vi "Apply Config.vi"(8 "error in (no error)":errorcluster, 11 "GaugeIndicator in":refnum<class "GaugeIndicator.lvclass">) -> (0 "error out":errorcluster, 3 "GaugeIndicator out":refnum<class "GaugeIndicator.lvclass">)   [LabVIEW 2020, in "VolatusGUIElements.lvlib" / "GaugeIndicator.lvclass"]
uses:
  GaugeIndicator.lvclass
  GaugeIndicator.lvclass/GaugeIndicator.ctl
  Value Source.ctl
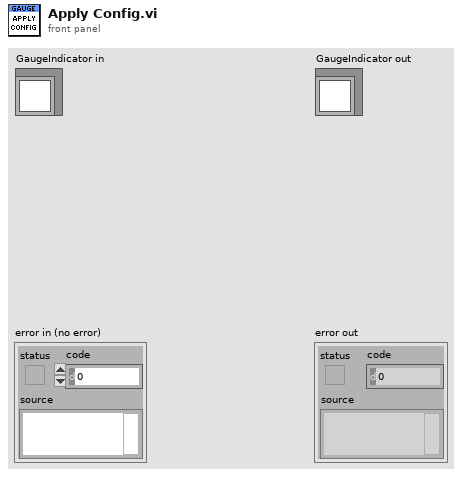
[diagram p1: front panel]
types:
  T1 = typedef "VolatusGUIElements.lvlib/GaugeIndicator.lvclass/Value Source.ctl" = enum16{"Constant", "Channel"}
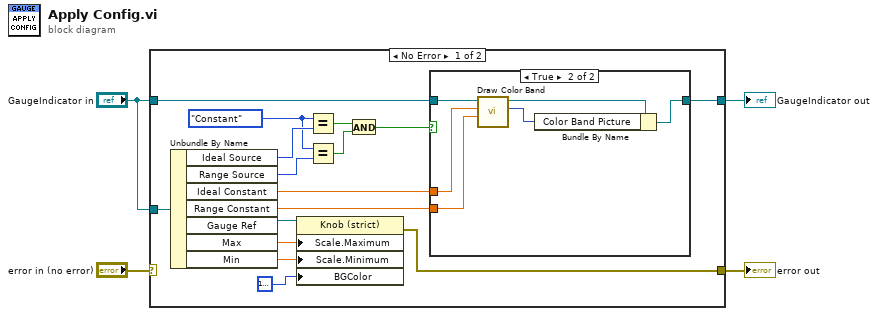
[diagram p0: block diagram]
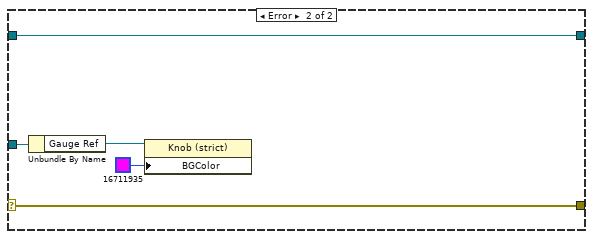
[diagram p3: hidden frame]
diagram:
  n1 = case shown="No Error" "error in (no error)" {
    selector: "error in (no error)" -> [_ w30]
    tunnel: "GaugeIndicator in" -> [w20 w32]
    tunnel: [w15 w30] -> w3
    tunnel: "GaugeIndicator in" -> [w9 w28]
    tunnel: [w5 w28] -> w1
    frame No Error {
      w12 = Value_Source."Constant" ("x")
      n2 = Unbundle By Name(w20) -> ("Ideal Source"=w14:T1, "Range Source"=w13:T1, "Ideal Constant"=w6:dbl, "Range Constant"=w7:dbl, "Gauge Ref"=w19:refnum<vi>, "Max"=w18:dbl, "Min"=w17:dbl)
      n3 = property class="Knob (strict)"(reference=w19, "Scale.Maximum"=w18, "Scale.Minimum"=w17, "BGColor"=u32 16777216 ("Housing Colors:BG Color")) -> (error out=w15:errorcluster)  [unwired: 1 in, 1 out]
      n4 = Equal?(x=w12, y=w14) -> (x = y?=w11:bool)
      n5 = Equal?(x=w12, y=w13) -> (x = y?=w10:bool)
      n6 = And(x=w11, y=w10) -> (x .and. y?=w8:bool)
      n7 = case shown="True" w8 {
        tunnel: w9 -> [w21 w27]
        tunnel: w7 -> [_ w25]
        tunnel: w6 -> [_ w26]
        tunnel: [w21 w22] -> w5
        frame False {
        }
        frame True {
          n8 = call "Draw Color Band.vi"("Range"=w25, "Ideal"=w26, "GaugeIndicator in"=w27) -> ("Color Band"=w23:picture, "GaugeIndicator out"=w24:refnum<class "GaugeIndicator.lvclass">)  [unwired: 6 in, 1 out]
          n9 = Bundle By Name(cluster=w24, "Color Band Picture"=w23) -> (w22:refnum<class "GaugeIndicator.lvclass">)
        }
      }
    }
    frame Error {
      n10 = Unbundle By Name(w32) -> ("Gauge Ref"=w31:refnum<vi>)
      n11 = property class="Knob (strict)"(reference=w31, "BGColor"=u32 16711935 ("Housing Colors:BG Color")) -> ()  [unwired: 1 in, 2 out]
    }
  }
  "error out" <- w3
  "GaugeIndicator out" <- w1
